vi "Menu Resolve Shortcut.vi"(0 "输入字符串":string) -> (1 "快捷方式":T1 caption="菜单快捷方式", 2 "项名称":string, 3 "项标识符":string)   [LabVIEW 2011]
uses:
  <vilib>/Utility/miscctls.llb/LVMenuShortCut.ctl
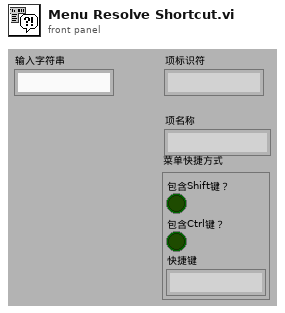
[diagram p1: front panel]
types:
  T1 = typedef "LVMenuShortCut.ctl" = cluster{"Include Shift Key?":bool, "Include Ctrl Key?":bool, "Shortcut Key":string}
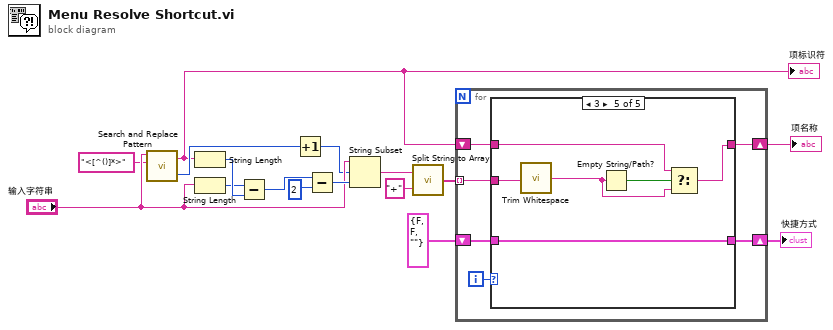
[diagram p0: block diagram]
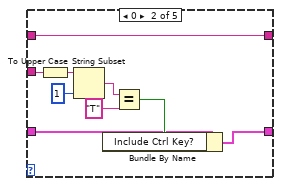
[diagram p3: hidden frame]
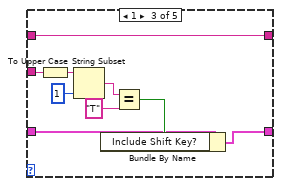
[diagram p4: hidden frame]
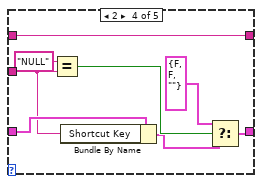
[diagram p5: hidden frame]
diagram:
  n1 = call <vilib>:"Search and Replace Pattern.vi"("string"="输入字符串", "regular expression (\"\")"="<[^()]*>" ("regular expression (\"\")")) -> ("result string"=w3:string, "offset past match"=w10:i32)  [unwired: 3 in]
  "项标识符" <- w3
  n2 = String Length(string=w3) -> (length=w13:i32)
  n3 = String Length(string="输入字符串") -> (length=w12:i32)
  n4 = Subtract(x=w12, y=w13) -> (x-y=w14:i32)
  n5 = Increment(x=w10) -> (x+1=w9:i32)
  n6 = Subtract(x=w14, y=2) -> (x-y=w16:i32)
  n7 = String Subset(string="输入字符串", offset (0)=w9, length (rest)=w16) -> (substring=w7:string)
  n8 = call "Split String to Array.vi"("搜索字符串/字符(-)"="+", "字符串"=w7) -> ("字符串数组"=w6:string[])
  n9 = for {
    tunnel: w6 -> [w19] mode=indexing
    shift-right: [w20] -> w4
    shift-left: T1 {"Include Shift Key?"=FALSE, "Include Ctrl Key?"=FALSE, "Shortcut Key"=""} ("快捷方式") -> [w21]
    shift-right: [w17] -> w2
    shift-left: w3 -> [w18]
    i -> [w22]
    n10 = case shown="3" w22 {
      tunnel: w21 -> [w24 w27 w36 w50 w56]
      tunnel: [w24 w26 w35 w47 w56] -> w20
      tunnel: w19 -> [_ w33 w42 w49 w52]
      tunnel: w18 -> [w23 w25 w34 w43 w54]
      tunnel: [w23 w25 w34 w43 w53] -> w17
      frame -1, Default {
      }
      frame 0 {
        n11 = To Upper Case(1:w33) -> (0:w32:string)
        n12 = String Subset(string=w32, length (rest)=1 ("长度（剩余）")) -> (substring=w30:string)  [unwired: 1 in]
        n13 = Equal?(x=w30, y="T") -> (x = y?=w28:bool)
        n14 = Bundle By Name(cluster=w27, "Include Ctrl Key?"=w28) -> (w26:T1)
      }
      frame 1 {
        n15 = To Upper Case(1:w42) -> (0:w41:string)
        n16 = String Subset(string=w41, length (rest)=1 ("长度（剩余）")) -> (substring=w39:string)  [unwired: 1 in]
        n17 = Equal?(x=w39, y="T") -> (x = y?=w37:bool)
        n18 = Bundle By Name(cluster=w36, "Include Shift Key?"=w37) -> (w35:T1)
      }
      frame 2 {
        n19 = Equal?(x="NULL", y=w49) -> (x = y?=w46:bool)
        n20 = Bundle By Name(cluster=w50, "Shortcut Key"=w49) -> (w44:T1)
        n21 = Select(t=T1 {"Include Shift Key?"=FALSE, "Include Ctrl Key?"=FALSE, "Shortcut Key"=""} ("快捷方式"), s=w46, f=w44) -> (s? t:f=w47:T1)
      }
      frame 3 {
        n22 = call <vilib>:"Trim Whitespace.vi"("string"=w52) -> ("trimmed string"=w51:string)  [unwired: 1 in]
        n23 = Empty String/Path?(string/path=w51) -> (empty?=w55:bool)
        n24 = Select(t=w54, s=w55, f=w51) -> (s? t:f=w53:string)
      }
    }
  }
  "项名称" <- w2
  "快捷方式" <- w4
